vi "Open.vi"(8 "error in":errorcluster, 9 "timeout (-1)":i32=-1, 11 "Standard Engine Runtime in":refnum<class "Standard Engine Runtime.lvclass">) -> (0 "error out":errorcluster, 3 "Standard Engine Runtime out":refnum<class "Standard Engine Runtime.lvclass">)   [LabVIEW 2013, in "Standard Engine Runtime.lvclass"]
doc: "This VI launches an engine background process that then waits for commands from the other API functions."
uses:
  Standard Engine Runtime.lvclass
  <vilib>/NI/Module Execution Interface/Engine Runtime/Execution States.ctl
  <vilib>/NI/Module Execution Interface/Engine Runtime/Fault.ctl
  <vilib>/NI/Tag Bus Module Framework/runtime/error classification.ctl
  main engine/engine references.ctl
  worker library/worker library reference.ctl
  worker library/worker comms.ctl
  worker library/worker commands.ctl
  worker library/request fifos.ctl
  worker library/recovery request.ctl
  <vilib>/NI/Tag Bus Module Framework/runtime/TBM module execution interface.lvclass
  <vilib>/NI/Tag Bus Module Framework/module configuration/TBM module configuration.lvclass
  worker library/rt fault.ctl
  worker library/response fifos.ctl
  worker library/recovery response.ctl
  Standard Engine Runtime.lvclass/Standard Engine Runtime.ctl
  async executor/async worker process.vi
  main engine/main engine.lvlib
  <vilib>/NI/Module Execution Interface/Engine Runtime/Engine Runtime Interface.lvclass
  worker library/worker pool.lvlib
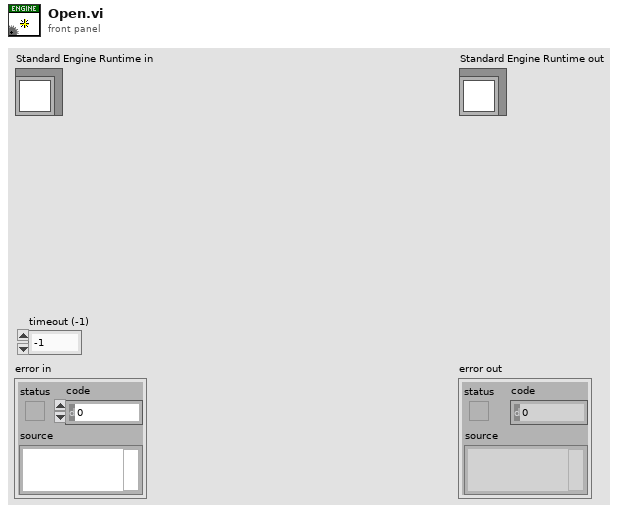
[diagram p1: front panel]
types:
  T1 = typedef "Engine Runtime Interface.lvclass/Execution States.ctl" = enum16{"Init", "Pre-Operational", "Safe-Operational", "Operational", "Stopped"}
  T2 = cluster{"read mode":enum16{"polling", "blocking"}, "write mode":enum16{"polling", "blocking"}}
  T3 = typedef "worker pool.lvlib/recovery response.ctl" = cluster{"module ref":refnum<data-value>, "engine reference":i32, "original run flags":u8, "success?":bool, "error code":i32}
  T4 = typedef "worker pool.lvlib/response fifos.ctl" = cluster{"recovery":refnum<k33>}
  T5 = typedef "main engine.lvlib/engine references.ctl" = cluster{"state notifier":refnum<notifier>, "Error Queue":refnum<queue>, "cmd fifo":refnum<k33>, "config DVR":refnum<data-value>, "worker pool":T6, "async exec pool":variant}
  T6 = typedef "worker pool.lvlib/worker library reference.ctl" = cluster{"vi ref":variant, "worker comms":T7, "worker count":i32}
  T7 = typedef "worker pool.lvlib/worker comms.ctl" = cluster{"command fifo":refnum<k33>, "request fifos":T8, "response fifos":T4, "fault list":refnum<data-value>}
  T8 = typedef "worker pool.lvlib/request fifos.ctl" = cluster{"recovery":refnum<k33>, "fault fifo":refnum<k33>}
  T9 = typedef "Engine Runtime Interface.lvclass/Fault.ctl" = cluster{"code":i32, "error classification":T10, "Source GUID":string, "first reported time":timestamp, "number reported":u32, "last reported time":timestamp}
  T10 = typedef "TBM module execution interface.lvclass/error classification.ctl" = enum16{"unknown", "none", "trivial", "recoverable", "critical"}
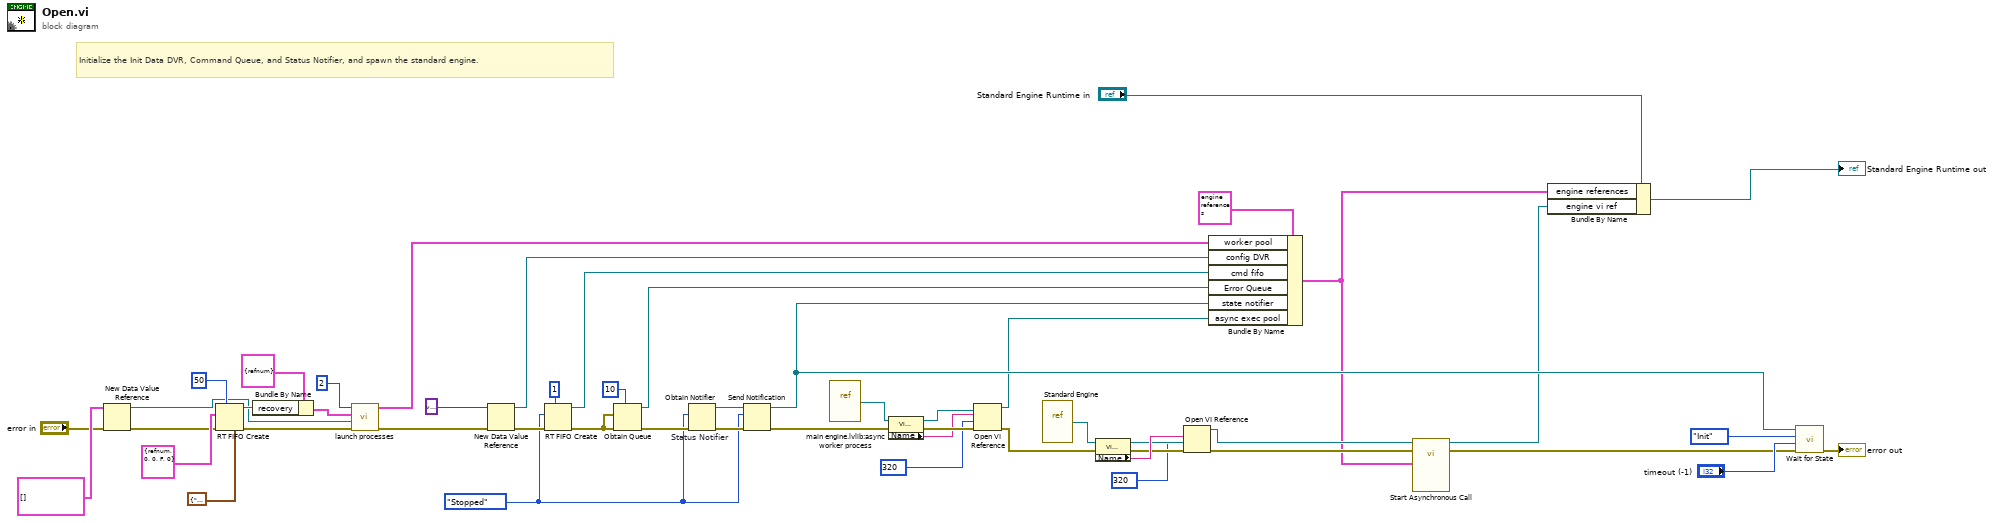
[diagram p0: block diagram]
diagram:
  w26 = Execution_States."Stopped" ("States")
  # "Initialize the Init Data DVR, Command Queue, and Status Notifier, and spawn the standard engine."
  n1 = New Data Value Reference(data value=T9[] [] ("faults"), error in="error in") -> (data value reference=w24:refnum<data-value>, error out=w25:errorcluster)
  n2 = RT FIFO Create(1:T3 {"module ref"=refnum, "engine reference"=0, "original run flags"=0, "success?"=FALSE, "error code"=0} ("recovery response"), 3:w25, 4:u32 50 ("size (10)"), 7:T2 {"read mode"=enum."polling", "write mode"=enum."blocking"} ("r/w modes (polling,polling)")) -> (8:w30:refnum<k33>, 11:w27:errorcluster)  [unwired: 4 in, 1 out]
  n3 = Bundle By Name(cluster=T4 {"recovery"=refnum} ("response fifos"), "recovery"=w30) -> (w29:T4)
  n4 = call "launch processes.vi"("error in"=w27, "fault list"=w24, "response fifos"=w29, "pool size"=u8 2) -> ("error out"=w23:errorcluster, "worker reference"=w21:T6)  [unwired: 6 in]
  n5 = New Data Value Reference ("Configuration Data")(data value=variant ("variant"), error in=w23) -> (data value reference=w20:refnum<data-value>, error out=w49:errorcluster)
  n6 = RT FIFO Create ("Messages FIFO")(1:w26, 3:w49, 4:u32 1 ("size (10)")) -> (8:w19:refnum<k33>, 11:w43:errorcluster)  [unwired: 5 in, 1 out]
  n7 = Obtain Queue(max queue size (-1, unlimited)=10, element data type=w43, error in (no error)=w43) -> (queue out=w18:refnum<queue>, error out=w45:errorcluster)  [unwired: 2 in, 1 out]
  n8 = Obtain Notifier "Status Notifier"(notification data type=w26, error in (no error)=w45) -> (notifier out=w46:refnum<notifier>, error out=w47:errorcluster)  [unwired: 2 in, 1 out]
  n9 = Send Notification(notification=w26, notifier=w46, error in (no error)=w47) -> (notifier out=w17:refnum<notifier>, error out=w5:errorcluster)
  n10 = vi-ref "main engine.lvlib:async worker process.vi"() -> (w1:refnum<vi>)
  n11 = property class="VI (strict)"(reference=w1, error in=w5) -> (reference out=w8:refnum<vi>, error out=w7:errorcluster, "Name"=w6:string)
  n12 = Open VI Reference(type specifier VI Refnum (for type only)=w8, vi path=w6, options=320, error in (no error)=w7) -> (vi reference=w2:refnum<vi>, error out=w3:errorcluster)  [unwired: 2 in]
  n13 = vi-ref "Standard Engine.vi"() -> (w48:refnum<vi>)
  n14 = property class="VI (strict)"(reference=w48, error in=w3) -> (reference out=w15:refnum<vi>, error out=w50:errorcluster, "Name"=w51:string)
  n15 = Open VI Reference(type specifier VI Refnum (for type only)=w15, vi path=w51, options=320, error in (no error)=w50) -> (vi reference=w10:refnum<vi>, error out=w13:errorcluster)  [unwired: 2 in]
  n16 = Bundle By Name(cluster=T5 {"state notifier"=refnum, "Error Queue"=refnum, "cmd fifo"=refnum, "config DVR"=refnum, "worker pool"={"vi ref"=variant, "worker comms"={"command fifo"=refnum, "request fifos"={"recovery"=refnum, "fault fifo"=refnum}, "response fifos"={"recovery"=refnum}, "fault list"=refnum}, "worker count"=0}, "async exec pool"=variant} ("engine references"), "worker pool"=w21, "config DVR"=w20, "cmd fifo"=w19, "Error Queue"=w18, "state notifier"=w17, "async exec pool"=w2) -> (w9:T5)
  n17 = call-by-ref "Start Asynchronous Call"(reference=w10, error in=w13, "engine references"=w9) -> (reference out=w11:refnum<vi>, error out=w12:errorcluster)  [unwired: 11 in]
  n18 = Bundle By Name(cluster="Standard Engine Runtime in", "engine references"=w9, "engine vi ref"=w11) -> (→"Standard Engine Runtime out":refnum<class "Standard Engine Runtime.lvclass">)
  n19 = call "Wait for State.vi"("error in"=w12, "timeout in ms"="timeout (-1)", "desired state"=Execution_States."Init", "state notifier"=w17) -> ("error out"=→"error out":errorcluster)  [unwired: 7 in]
